vi "worker_go.vi"() -> ()   [LabVIEW 2015]
panel:
  in  "Number of workers":i32=5
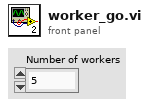
[diagram p1: front panel]
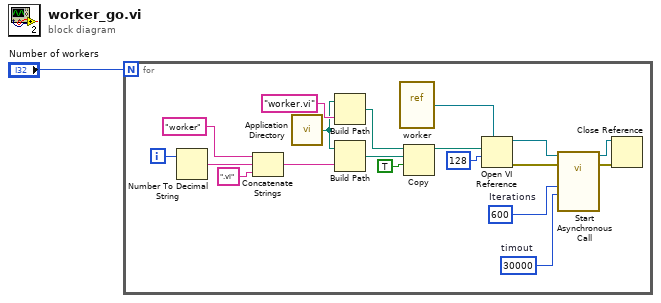
[diagram p0: block diagram]
diagram:
  n1 = for {
    N: "Number of workers" -> [_]
    i -> [w4]
    w2 = 30000  # timout
    w3 = 600  # Iterations
    n2 = Number To Decimal String(number=w4) -> (decimal integer string=w16:string)  [unwired: 1 in]
    n3 = Concatenate Strings("worker" ("string"), w16, ".vi" ("string")) -> (w14:string)
    n4 = call <vilib>:"Application Directory.vi"() -> ("Application Directory"=w18:path)
    n5 = Build Path(base path=w18, name or relative path="worker.vi") -> (appended path=w19:path)
    n6 = Build Path(base path=w18, name or relative path=w14) -> (appended path=w13:path)
    n7 = vi-ref "worker.vi"() -> (w11:refnum<vi>)
    n8 = Copy(9:TRUE ("overwrite (F)"), 10:w13, 11:w19) -> (3:w10:path)  [unwired: 2 in, 2 out]
    n9 = Open VI Reference(type specifier VI Refnum (for type only)=w11, vi path=w10, options=128) -> (vi reference=w9:refnum<vi>, error out=w5:errorcluster)  [unwired: 3 in]
    n10 = call-by-ref "Start Asynchronous Call"(reference=w9, error in=w5, "timout"=w2, "Iterations"=w3) -> (reference out=w6:refnum<vi>, error out=w7:errorcluster)  [unwired: 10 in]
    n11 = Close Reference(reference=w6, error in (no error)=w7) -> ()  [unwired: 1 out]
  }
